vi "DBL.vi"(4 "Value":T1) -> (1 "Constant":refnum<class "Const_EXT.lvclass">)   [LabVIEW 2021, in "Const_EXT.lvclass"]
uses:
  Const_EXT.lvclass
  Type.ctl
  Const_EXT.lvclass/Const_EXT.ctl
  Properties/Write Value.vi
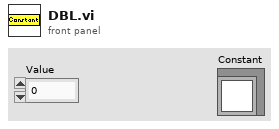
[diagram p1: front panel]
types:
  T1 = typedef "Const_EXT.lvclass/Type.ctl" = dbl
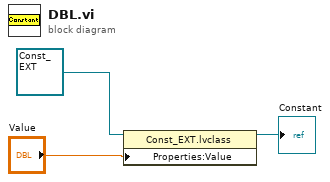
[diagram p0: block diagram]
diagram:
  n1 = property class="Const_EXT.lvclass"(reference=refnum<class "Const_EXT.lvclass"> refnum ("Constants.lvlib:Numeric.lvclass"), "Properties:Value"="Value") -> (reference out=→"Constant":refnum<class "Const_EXT.lvclass">)  [unwired: 1 in, 1 out]
